vi "Handle.vi"(8 "error in (no error)":errorcluster, 11 "Sync Box in":refnum<class "Sync Box.lvclass">) -> (0 "error out":errorcluster, 3 "Sync Box out":refnum<class "Sync Box.lvclass">)   [LabVIEW 2018, in "Sync Box.lvclass"]
uses:
  Sync Box.lvclass
  Sync Box.lvclass/Sync Box.ctl
  Device/Device.lvclass/Device.ctl
  Trigger/Trigger.lvclass
  C:/Users/observer/Desktop/Sparc4GUI/SPARC4_GUI/Device/Device.lvclass
  Server/Server.lvclass
  Comm/Stream/Stream.lvclass
  Device/Device.lvclass
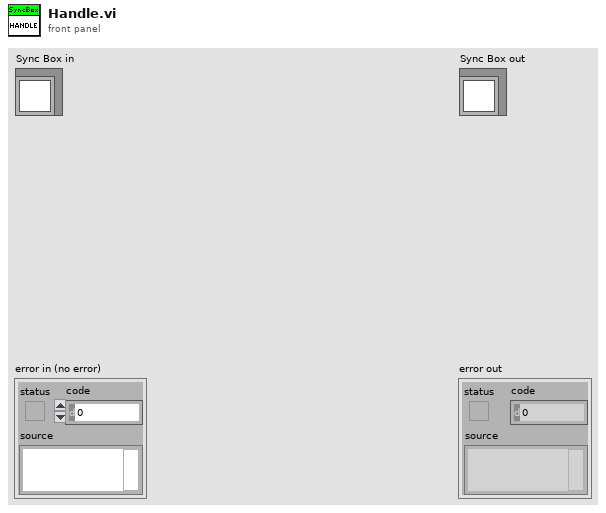
[diagram p1: front panel]
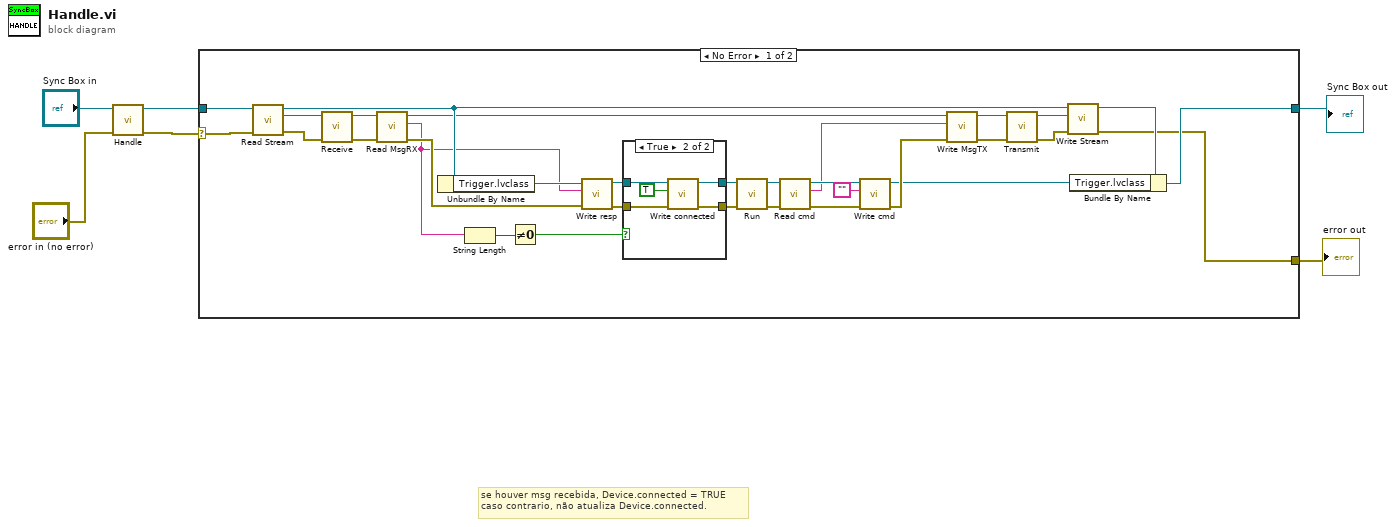
[diagram p0: block diagram]
diagram:
  # "se houver msg recebida, Device.connected = TRUE\ncaso contrario, não atualiza Device.connected."
  n1 = call-parent "Handle.vi"("error in (no error)"="error in (no error)", "Server in"="Sync Box in") -> ("error out"=w3:errorcluster, "Server out"=w4:refnum<class "Sync Box.lvclass">)  [unwired: 8 in]
  n2 = case shown="No Error" w3 {
    selector: w3 -> [w36 w47]
    tunnel: [w25 w47] -> w1
    tunnel: [w35 w46] -> w2
    tunnel: w4 -> [w24 w46]
    frame No Error {
      n3 = call-dynamic "Read Stream.vi"("error in (no error)"=w36, "Server in"=w24) -> ("error out"=w37:errorcluster, "Stream.lvclass"=w38:refnum<class "Stream.lvclass">, "Server out"=w28:refnum<class "Sync Box.lvclass">)  [unwired: 7 in]
      n4 = call-dynamic "Receive.vi"("error in (no error)"=w37, "Stream in"=w38) -> ("error out"=w34:errorcluster, "Stream out"=w33:refnum<class "Stream.lvclass">)  [unwired: 8 in]
      n5 = call-dynamic "Read MsgRX.vi"("error in (no error)"=w34, "Comm in"=w33) -> ("error out"=w32:errorcluster, "MsgRX"=w15:string, "Comm out"=w16:refnum<class "Stream.lvclass">)  [unwired: 7 in]
      n6 = Unbundle By Name(w28) -> ("Trigger.lvclass"=w20:refnum<class "Trigger.lvclass">)
      n7 = String Length(string=w15) -> (length=w7:i32)
      n8 = Not Equal To 0?(x=w7) -> (x != 0?=w12:bool)
      n9 = call-dynamic "Write resp.vi"("error in (no error)"=w32, "resp"=w15, "Device in"=w20) -> ("error out"=w10:errorcluster, "Device out"=w11:refnum<class "Trigger.lvclass">)  [unwired: 7 in]
      n10 = case shown="True" w12 {
        tunnel: w10 -> [w39 w45]
        tunnel: w11 -> [w40 w44]
        tunnel: [w40 w43] -> w8
        tunnel: [w39 w42] -> w9
        frame False {
        }
        frame True {
          n11 = call "Write connected.vi"("error in (no error)"=w45, "connected"=TRUE, "Device in"=w44) -> ("error out"=w42:errorcluster, "Device out"=w43:refnum<class "Trigger.lvclass">)  [unwired: 7 in]
        }
      }
      n12 = call-dynamic "Run.vi"("error in (no error)"=w9, "Trigger in"=w8) -> ("error out"=w13:errorcluster, "Trigger out"=w14:refnum<class "Trigger.lvclass">)  [unwired: 8 in]
      n13 = call-dynamic "Read cmd.vi"("error in (no error)"=w13, "Device in"=w14) -> ("error out"=w22:errorcluster, "cmd"=w18:string, "Device out"=w23:refnum<class "Trigger.lvclass">)  [unwired: 7 in]
      n14 = call-dynamic "Write cmd.vi"("error in (no error)"=w22, "cmd"="", "Device in"=w23) -> ("error out"=w31:errorcluster, "Device out"=w19:refnum<class "Trigger.lvclass">)  [unwired: 7 in]
      n15 = call-dynamic "Write MsgTX.vi"("error in (no error)"=w31, "MsgTX"=w18, "Comm in"=w16) -> ("error out"=w29:errorcluster, "Comm out"=w30:refnum<class "Stream.lvclass">)  [unwired: 7 in]
      n16 = call-dynamic "Transmit.vi"("error in (no error)"=w29, "Stream in"=w30) -> ("error out"=w26:errorcluster, "Stream out"=w17:refnum<class "Stream.lvclass">)  [unwired: 8 in]
      n17 = call-dynamic "Write Stream.vi"("error in (no error)"=w26, "Stream.lvclass"=w17, "Server in"=w28) -> ("error out"=w25:errorcluster, "Server out"=w27:refnum<class "Sync Box.lvclass">)  [unwired: 7 in]
      n18 = Bundle By Name(cluster=w27, "Trigger.lvclass"=w19) -> (w35:refnum<class "Sync Box.lvclass">)
    }
    frame Error {
    }
  }
  "error out" <- w1
  "Sync Box out" <- w2
